vi "write_ini.vi"(8 "error in (no error)":errorcluster caption="错误输入（无错误）", 9 "section name":string, 10 "file ref in":T1, 11 "StepMotor 输入":refnum<class "StepMotor.lvclass">) -> (0 "error out":errorcluster caption="错误输出", 2 "file ref out":T1, 3 "StepMotor 输出":refnum<class "StepMotor.lvclass">)   [LabVIEW 2016, in "MotionControl_UFO_3DOF.lvlib" / "StepMotor.lvclass"]
uses:
  <userlib>/MotionControl_UFO_3DOF/StepMotor/StepMotor.lvclass
  <vilib>/Utility/config.llb/Config Data RefNum.ctl
  <userlib>/MotionControl_UFO_3DOF/StepMotor/StepMotor.lvclass/StepMotor.ctl
  <vilib>/Utility/config.llb/Write Key (U32).vi
  <vilib>/Utility/config.llb/Write Key (I32).vi
  <vilib>/Utility/config.llb/Write Key (Double).vi
  <vilib>/Utility/config.llb/Write Key (Boolean).vi
  <vilib>/Utility/error.llb/Error Cluster From Error Code.vi
  <vilib>/ErrorRing/Error Ring.xnode
  <vilib>/Utility/config.llb/NI_LVConfig.lvlib
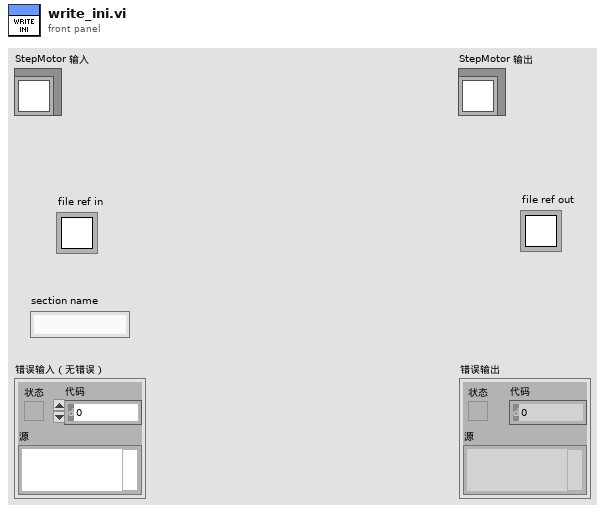
[diagram p1: front panel]
types:
  T1 = typedef "NI_LVConfig.lvlib/Config Data RefNum.ctl" = refnum<k1>
  T2 = typedef "MotionControl_UFO_3DOF.lvlib/StepMotor.lvclass/AdvMovePara.ctl" = cluster{"acceleration":i32, "deceleration":i32, "max startup speed":i32, "max stop speed":i32}
  T3 = typedef "MotionControl_UFO_3DOF.lvlib/StepMotor.lvclass/UIM_ICFG.ctl" = cluster{"ENA-开机自动使能":bool, "CCW-设置电机正转向":bool, "UPG-上电自动执行用户程序":bool, "ELOCK-紧急上锁功能":bool, "S1C-开机使能S1":bool, "S2C-开机使能S2":bool, "S3C-开机使能S3":bool, "S4C-开机使能S4":bool}
  T4 = typedef "MotionControl_UFO_3DOF.lvlib/StepMotor.lvclass/UIM_MCFG.ctl" = cluster{"bS1IE":bool, "bS2IE":bool, "bS3IE":bool, "bP4IE":bool, "bSTPIE":bool, "bORGIE":bool, "bSTLIE":bool, "bDM":bool, "bAM":bool, "bCM":bool, "bQEM":bool, "bQEI":bool, "bCHS":bool, "bANE":bool}
  T5 = typedef "MotionControl_UFO_3DOF.lvlib/StepMotor.lvclass/S12CON.ctl" = cluster{"S2传感器上升沿绑定动作":u32, "S2传感器下降沿绑定动作":u32, "S1传感器上升沿绑定动作":u32, "S1传感器下降沿绑定动作":u32}
  T6 = typedef "MotionControl_UFO_3DOF.lvlib/StepMotor.lvclass/S34CON.ctl" = cluster{"TRUE: P4 出低电平; FALSE: P4 出高电平。":bool, "P4输出关联的事件代码":u32, "S3传感器上升沿绑定动作":u32, "S3传感器下降沿绑定动作":u32, "当发生堵转时动作":u32}
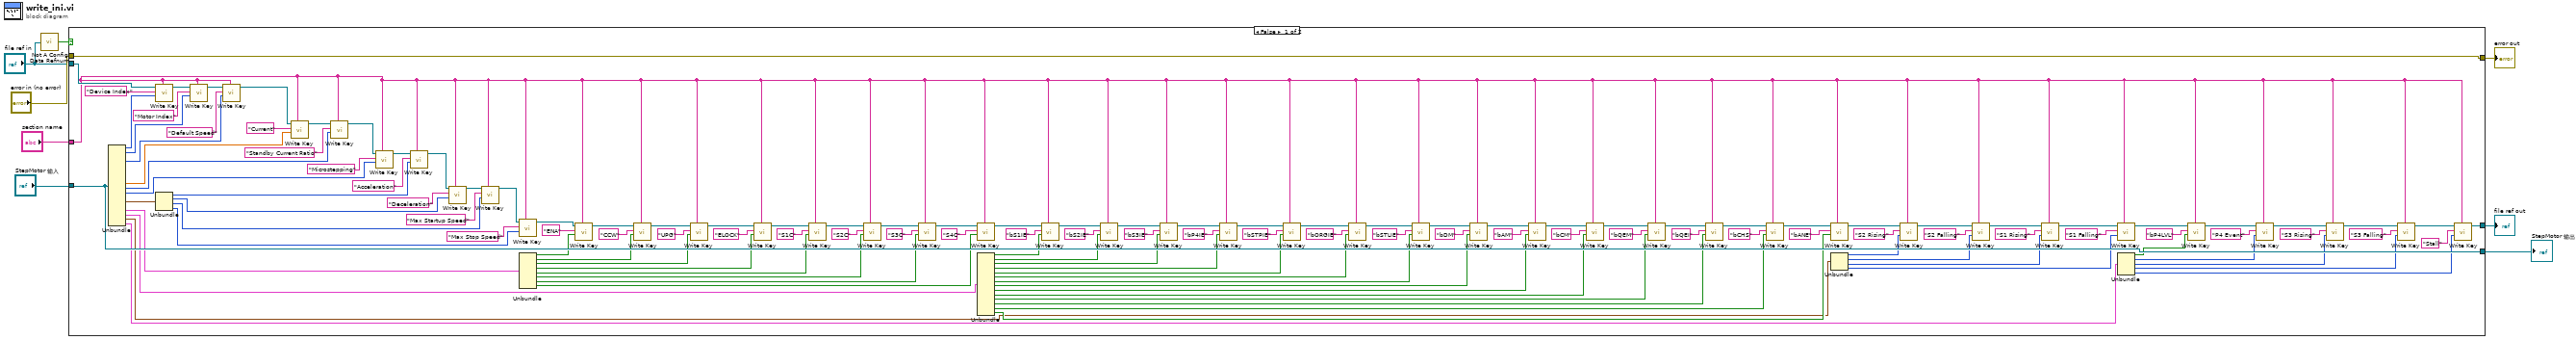
[diagram p0: block diagram]
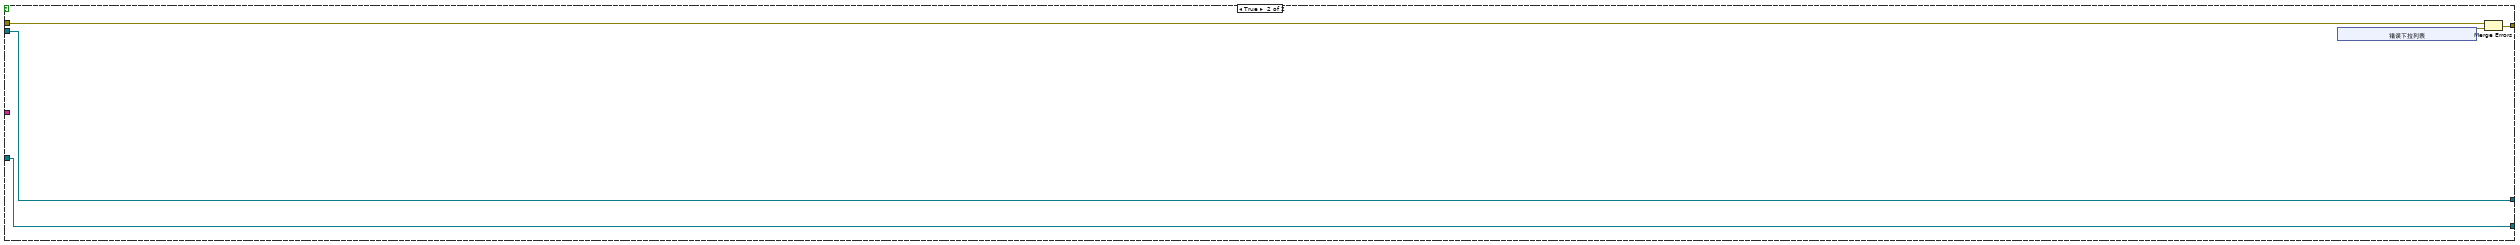
[diagram p2: hidden frame]
diagram:
  n1 = call <vilib>:"Not A Config Data Refnum.vi"("refnum"="file ref in") -> ("not a config data refnum"=w5:bool)
  n2 = case shown="False" w5 {
    tunnel: [w140 w141] -> w8
    tunnel: [w138 w145] -> w6
    tunnel: "StepMotor 输入" -> [w138 w145]
    tunnel: "error in (no error)" -> [w140 w142]
    tunnel: [w9 w144] -> w3
    tunnel: "file ref in" -> [w114 w144]
    tunnel: "section name" -> [w20 _]
    frame False {
      n3 = Unbundle(w138) -> (w109:u32, w108:u32, w137:i32, w134:dbl, w129:i32, w128:u32, w125:T2, w91:T3, w55:T4, w24:T5, w23:T6)  [unwired: 7 out]
      n4 = call-poly <vilib>:"Write Key.vi"("section"=w20, "value"=w109, "key"="Device Index", "refnum"=w114) -> ("refnum out"=w113:T1)  [unwired: 5 in, 2 out]
      n5 = Unbundle(w125) -> ("acceleration"=w124:i32, "deceleration"=w118:i32, "max startup speed"=w117:i32, "max stop speed"=w115:i32)
      n6 = call-poly <vilib>:"Write Key.vi"("section"=w20, "value"=w108, "key"="Motor Index", "refnum"=w113) -> ("refnum out"=w112:T1)  [unwired: 5 in, 2 out]
      n7 = call-poly <vilib>:"Write Key.vi"("section"=w20, "value"=w137, "key"="Default Speed", "refnum"=w112) -> ("refnum out"=w136:T1)  [unwired: 5 in, 2 out]
      n8 = call-poly <vilib>:"Write Key.vi"("section"=w20, "value"=w134, "key"="Current", "refnum"=w136) -> ("refnum out"=w132:T1)  [unwired: 5 in, 2 out]
      n9 = call-poly <vilib>:"Write Key.vi"("section"=w20, "value"=w129, "key"="Standby Current Ratio", "refnum"=w132) -> ("refnum out"=w130:T1)  [unwired: 5 in, 2 out]
      n10 = call-poly <vilib>:"Write Key.vi"("section"=w20, "value"=w128, "key"="Microstepping", "refnum"=w130) -> ("refnum out"=w127:T1)  [unwired: 5 in, 2 out]
      n11 = call-poly <vilib>:"Write Key.vi"("section"=w20, "value"=w124, "key"="Acceleration", "refnum"=w127) -> ("refnum out"=w123:T1)  [unwired: 5 in, 2 out]
      n12 = call-poly <vilib>:"Write Key.vi"("section"=w20, "value"=w118, "key"="Deceleration", "refnum"=w123) -> ("refnum out"=w122:T1)  [unwired: 5 in, 2 out]
      n13 = call-poly <vilib>:"Write Key.vi"("section"=w20, "value"=w117, "key"="Max Startup Speed", "refnum"=w122) -> ("refnum out"=w121:T1)  [unwired: 5 in, 2 out]
      n14 = call-poly <vilib>:"Write Key.vi"("section"=w20, "value"=w115, "key"="Max Stop Speed", "refnum"=w121) -> ("refnum out"=w92:T1)  [unwired: 5 in, 2 out]
      n15 = Unbundle(w91) -> ("ENA-开机自动使能"=w90:bool, "CCW-设置电机正转向"=w89:bool, "UPG-上电自动执行用户程序"=w88:bool, "ELOCK-紧急上锁功能"=w87:bool, "S1C-开机使能S1"=w86:bool, "S2C-开机使能S2"=w85:bool, "S3C-开机使能S3"=w84:bool, "S4C-开机使能S4"=w83:bool)
      n16 = call-poly <vilib>:"Write Key.vi"("section"=w20, "value"=w90, "key"="ENA", "refnum"=w92) -> ("refnum out"=w103:T1)  [unwired: 5 in, 2 out]
      n17 = call-poly <vilib>:"Write Key.vi"("section"=w20, "value"=w89, "key"="CCW", "refnum"=w103) -> ("refnum out"=w102:T1)  [unwired: 5 in, 2 out]
      n18 = call-poly <vilib>:"Write Key.vi"("section"=w20, "value"=w88, "key"="UPG", "refnum"=w102) -> ("refnum out"=w101:T1)  [unwired: 5 in, 2 out]
      n19 = call-poly <vilib>:"Write Key.vi"("section"=w20, "value"=w87, "key"="ELOCK", "refnum"=w101) -> ("refnum out"=w93:T1)  [unwired: 5 in, 2 out]
      n20 = call-poly <vilib>:"Write Key.vi"("section"=w20, "value"=w86, "key"="S1C", "refnum"=w93) -> ("refnum out"=w96:T1)  [unwired: 5 in, 2 out]
      n21 = call-poly <vilib>:"Write Key.vi"("section"=w20, "value"=w85, "key"="S2C", "refnum"=w96) -> ("refnum out"=w95:T1)  [unwired: 5 in, 2 out]
      n22 = call-poly <vilib>:"Write Key.vi"("section"=w20, "value"=w84, "key"="S3C", "refnum"=w95) -> ("refnum out"=w94:T1)  [unwired: 5 in, 2 out]
      n23 = call-poly <vilib>:"Write Key.vi"("section"=w20, "value"=w83, "key"="S4C", "refnum"=w94) -> ("refnum out"=w53:T1)  [unwired: 5 in, 2 out]
      n24 = Unbundle(w55) -> ("bS1IE"=w54:bool, "bS2IE"=w52:bool, "bS3IE"=w51:bool, "bP4IE"=w50:bool, "bSTPIE"=w49:bool, "bORGIE"=w48:bool, "bSTLIE"=w47:bool, "bDM"=w46:bool, "bAM"=w45:bool, "bCM"=w44:bool, "bQEM"=w43:bool, "bQEI"=w42:bool, "bCHS"=w41:bool, "bANE"=w40:bool)
      n25 = call-poly <vilib>:"Write Key.vi"("section"=w20, "value"=w54, "key"="bS1IE", "refnum"=w53) -> ("refnum out"=w78:T1)  [unwired: 5 in, 2 out]
      n26 = call-poly <vilib>:"Write Key.vi"("section"=w20, "value"=w52, "key"="bS2IE", "refnum"=w78) -> ("refnum out"=w77:T1)  [unwired: 5 in, 2 out]
      n27 = call-poly <vilib>:"Write Key.vi"("section"=w20, "value"=w51, "key"="bS3IE", "refnum"=w77) -> ("refnum out"=w76:T1)  [unwired: 5 in, 2 out]
      n28 = call-poly <vilib>:"Write Key.vi"("section"=w20, "value"=w50, "key"="bP4IE", "refnum"=w76) -> ("refnum out"=w58:T1)  [unwired: 5 in, 2 out]
      n29 = call-poly <vilib>:"Write Key.vi"("section"=w20, "value"=w49, "key"="bSTPIE", "refnum"=w58) -> ("refnum out"=w71:T1)  [unwired: 5 in, 2 out]
      n30 = call-poly <vilib>:"Write Key.vi"("section"=w20, "value"=w48, "key"="bORGIE", "refnum"=w71) -> ("refnum out"=w70:T1)  [unwired: 5 in, 2 out]
      n31 = call-poly <vilib>:"Write Key.vi"("section"=w20, "value"=w47, "key"="bSTLIE", "refnum"=w70) -> ("refnum out"=w69:T1)  [unwired: 5 in, 2 out]
      n32 = call-poly <vilib>:"Write Key.vi"("section"=w20, "value"=w46, "key"="bDM", "refnum"=w69) -> ("refnum out"=w57:T1)  [unwired: 5 in, 2 out]
      n33 = call-poly <vilib>:"Write Key.vi"("section"=w20, "value"=w45, "key"="bAM", "refnum"=w57) -> ("refnum out"=w64:T1)  [unwired: 5 in, 2 out]
      n34 = call-poly <vilib>:"Write Key.vi"("section"=w20, "value"=w44, "key"="bCM", "refnum"=w64) -> ("refnum out"=w63:T1)  [unwired: 5 in, 2 out]
      n35 = call-poly <vilib>:"Write Key.vi"("section"=w20, "value"=w43, "key"="bQEM", "refnum"=w63) -> ("refnum out"=w62:T1)  [unwired: 5 in, 2 out]
      n36 = call-poly <vilib>:"Write Key.vi"("section"=w20, "value"=w42, "key"="bQEI", "refnum"=w62) -> ("refnum out"=w56:T1)  [unwired: 5 in, 2 out]
      n37 = call-poly <vilib>:"Write Key.vi"("section"=w20, "value"=w41, "key"="bCHS", "refnum"=w56) -> ("refnum out"=w59:T1)  [unwired: 5 in, 2 out]
      n38 = call-poly <vilib>:"Write Key.vi"("section"=w20, "value"=w40, "key"="bANE", "refnum"=w59) -> ("refnum out"=w25:T1)  [unwired: 5 in, 2 out]
      n39 = Unbundle(w24) -> ("S2传感器上升沿绑定动作"=w19:u32, "S2传感器下降沿绑定动作"=w18:u32, "S1传感器上升沿绑定动作"=w17:u32, "S1传感器下降沿绑定动作"=w16:u32)
      n40 = call-poly <vilib>:"Write Key.vi"("section"=w20, "value"=w19, "key"="S2 Rising", "refnum"=w25) -> ("refnum out"=w35:T1)  [unwired: 5 in, 2 out]
      n41 = call-poly <vilib>:"Write Key.vi"("section"=w20, "value"=w18, "key"="S2 Falling", "refnum"=w35) -> ("refnum out"=w34:T1)  [unwired: 5 in, 2 out]
      n42 = call-poly <vilib>:"Write Key.vi"("section"=w20, "value"=w17, "key"="S1 Rising", "refnum"=w34) -> ("refnum out"=w33:T1)  [unwired: 5 in, 2 out]
      n43 = call-poly <vilib>:"Write Key.vi"("section"=w20, "value"=w16, "key"="S1 Falling", "refnum"=w33) -> ("refnum out"=w15:T1)  [unwired: 5 in, 2 out]
      n44 = Unbundle(w23) -> ("TRUE: P4 出低电平; FALSE: P4 出高电平。"=w14:bool, "P4输出关联的事件代码"=w13:u32, "S3传感器上升沿绑定动作"=w12:u32, "S3传感器下降沿绑定动作"=w11:u32, "当发生堵转时动作"=w10:u32)
      n45 = call-poly <vilib>:"Write Key.vi"("section"=w20, "value"=w14, "key"="bP4LVL", "refnum"=w15) -> ("refnum out"=w28:T1)  [unwired: 5 in, 2 out]
      n46 = call-poly <vilib>:"Write Key.vi"("section"=w20, "value"=w13, "key"="P4 Event", "refnum"=w28) -> ("refnum out"=w27:T1)  [unwired: 5 in, 2 out]
      n47 = call-poly <vilib>:"Write Key.vi"("section"=w20, "value"=w12, "key"="S3 Rising", "refnum"=w27) -> ("refnum out"=w26:T1)  [unwired: 5 in, 2 out]
      n48 = call-poly <vilib>:"Write Key.vi"("section"=w20, "value"=w11, "key"="S3 Falling", "refnum"=w26) -> ("refnum out"=w21:T1)  [unwired: 5 in, 2 out]
      n49 = call-poly <vilib>:"Write Key.vi"("section"=w20, "value"=w10, "key"="Stall", "refnum"=w21) -> ("refnum out"=w9:T1)  [unwired: 5 in, 2 out]
    }
    frame True {
      n50 = xnode "错误下拉列表"() -> ("error out"=w143:errorcluster)
      n51 = Merge Errors(w142, w143) -> (w141:errorcluster)
    }
  }
  "error out" <- w8
  "StepMotor 输出" <- w6
  "file ref out" <- w3
